vi "Write CS Logic Level.vi"(8 "error in (no error)":errorcluster, 10 "CS Logic Level":T1, 11 "LINX SPI in":refnum<class "LINX SPI.lvclass">) -> (0 "error out":errorcluster, 3 "LINX SPI out":refnum<class "LINX SPI.lvclass">)   [LabVIEW 2020, in "LINX SPI.lvclass"]
uses:
  LINX SPI.lvclass
  <vilib>/MakerHub/LINX/Private/Type Defs/Peripherals/SPI/SPI CS Logic Level.ctl
  <vilib>/MakerHub/LINX/LMH-LINX.lvlib
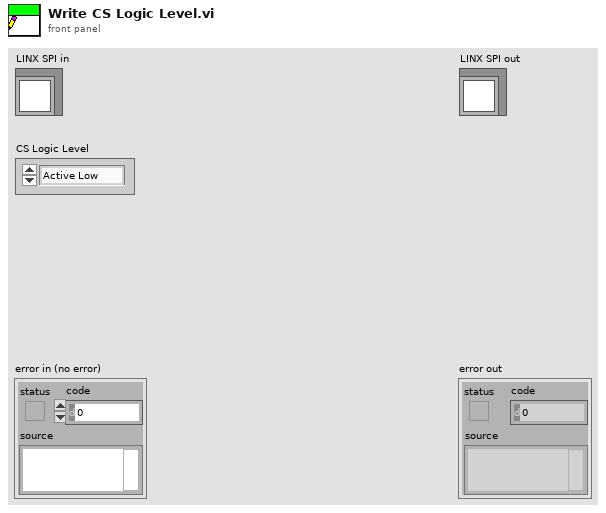
[diagram p1: front panel]
types:
  T1 = typedef "LMH-LINX.lvlib/SPI CS Logic Level.ctl" = enum8{"Active Low", "Active High"}
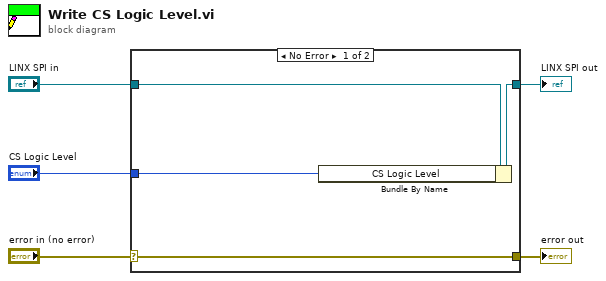
[diagram p0: block diagram]
diagram:
  n1 = case shown="No Error" "error in (no error)" {
    selector: "error in (no error)" -> [w9 w10]
    tunnel: [w9 w10] -> w4
    tunnel: [w7 w11] -> w2
    tunnel: "LINX SPI in" -> [w8 w11]
    tunnel: "CS Logic Level" -> [w6 _]
    frame No Error {
      n2 = Bundle By Name(cluster=w8, "CS Logic Level"=w6) -> (w7:refnum<class "LINX SPI.lvclass">)
    }
    frame Error {
    }
  }
  "error out" <- w4
  "LINX SPI out" <- w2
